vi "CAPFM-Acquire.vi"(0 "Runtime":T2, 11 "error in (no error)":errorcluster, 13 "Refs":T1) -> (6 "Control":dbl[](array[numeric]), 8 "Masked":dbl[](array[numeric]), 15 "error out":errorcluster)   [LabVIEW 2020]
uses:
  Typedefs/CAPFM-Runtime Data.ctl
  Typedefs/CAPFM-Control References.ctl
  <vilib>/Analysis/baseanly.llb/Mean (DBL).vi
  epl-vi-lib/Utility VIs/Conversion VIs/Create Waveform Cluster (2D).vi
  <vilib>/Analysis/NI_AALBase.lvlib
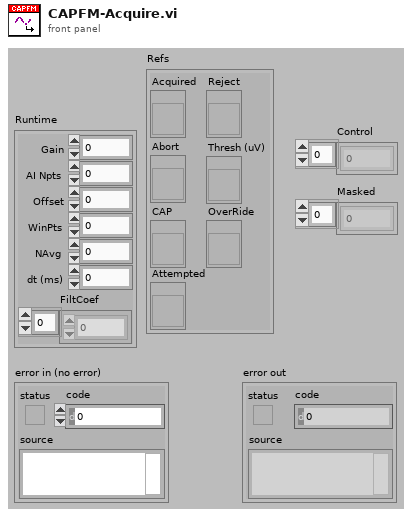
[diagram p1: front panel]
types:
  T1 = typedef "CAPFM-Control References.ctl" = cluster{"Acquired":refnum<vi>, "Abort":refnum<vi>, "CAP":refnum<vi>, "Reject":refnum<vi>, "Thresh (uV)":refnum<vi>, "OverRide":refnum<vi>, "Attempted":refnum<vi>}
  T2 = typedef "CAPFM-Runtime Data.ctl" = cluster{"Offset":i32, "AI Npts":i32, "Gain":dbl, "WinPts":i32, "NAvg":i32, "dt (ms)":dbl, "FiltCoef":dbl[]}
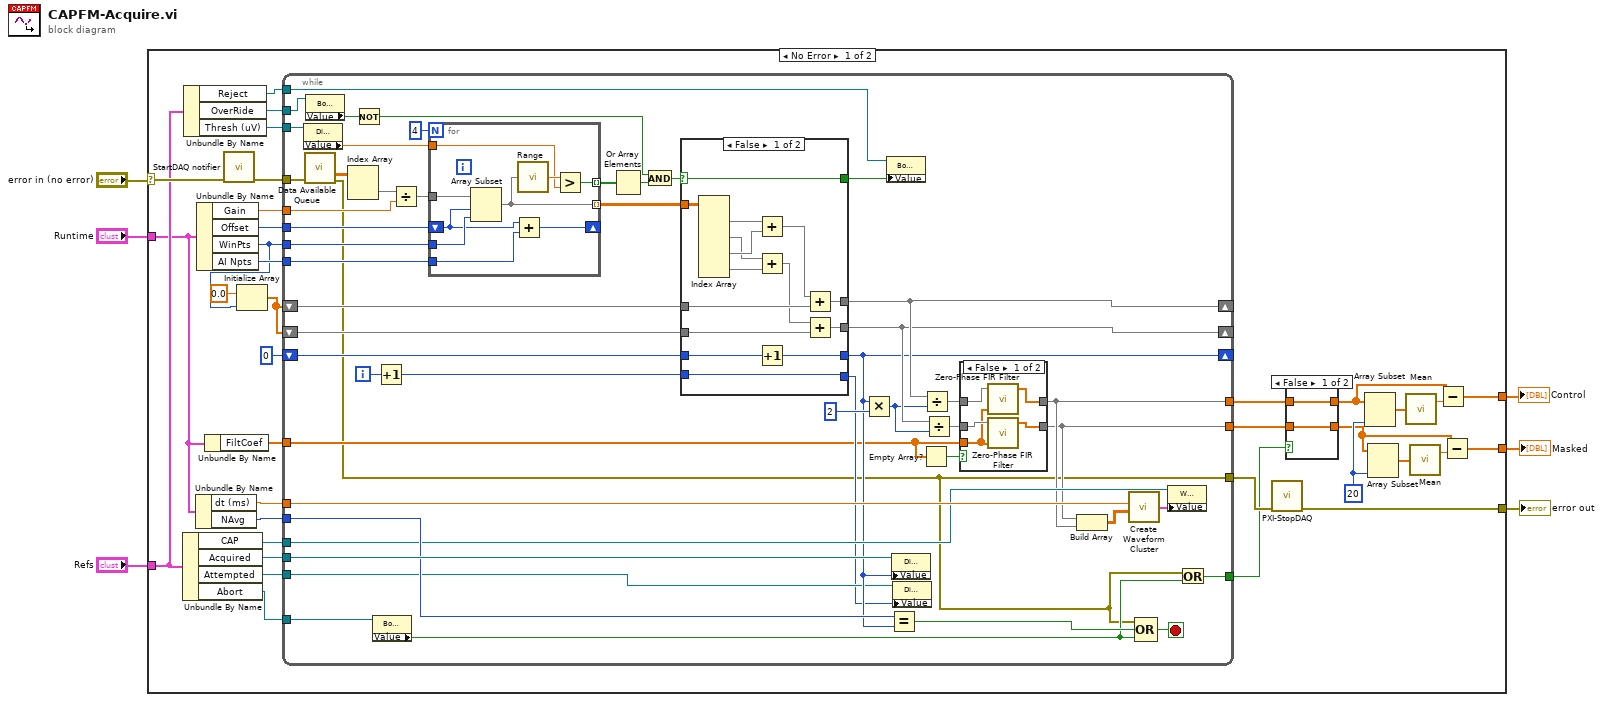
[diagram p0: block diagram]
diagram:
  n1 = case shown="No Error" "error in (no error)" {
    selector: "error in (no error)" -> [w41 w130]
    tunnel: [w29 w130] -> w5
    tunnel: "Runtime" -> [w8 _]
    tunnel: "Refs" -> [w22 _]
    tunnel: [w10 _] -> w2
    tunnel: [w9 _] -> w1
    frame No Error {
      w17 = 20
      n2 = Unbundle By Name(w22) -> ("CAP"=w31:refnum<vi>, "Acquired"=w35:refnum<vi>, "Attempted"=w19:refnum<vi>, "Abort"=w33:refnum<vi>)
      n3 = Unbundle By Name(w22) -> ("Reject"=w18:refnum<vi>, "OverRide"=w20:refnum<vi>, "Thresh (uV)"=w21:refnum<vi>)
      n4 = Unbundle By Name(w8) -> ("dt (ms)"=w32:dbl, "NAvg"=w34:i32)
      n5 = Unbundle By Name(w8) -> ("Gain"=w39:dbl, "Offset"=w37:i32, "WinPts"=w26:i32, "AI Npts"=w38:i32)
      n6 = Unbundle By Name(w8) -> ("FiltCoef"=w7:dbl[])
      n7 = call "StartDAQ notifier.vi"("error in (no error)"=w41) -> ("error out"=w40:errorcluster)  [unwired: 6 in]
      n8 = Initialize Array(0.0 ("element"), w26) -> (w28:dbl[])
      n9 = while {
        tunnel: w40 -> [w93]
        tunnel: w39 -> [w90]
        tunnel: w26 -> [w87]
        tunnel: w38 -> [w86]
        tunnel: w37 -> [w85]
        shift-right: [w75] -> _
        shift-left: w28 -> [w83]
        shift-right: [w74] -> _
        shift-left: w28 -> [w82]
        shift-right: [w57] -> _
        shift-left: 0 -> [w58]
        tunnel: w35 -> [w80]
        tunnel: w34 -> [w79]
        tunnel: w33 -> [w76]
        tunnel: w32 -> [w72]
        tunnel: w31 -> [w71]
        tunnel: [w46] -> w23
        tunnel: [w45] -> w24
        tunnel: [w44] -> w30
        tunnel: [w67] -> w25
        tunnel: w21 -> [w66]
        tunnel: w20 -> [w61]
        tunnel: w19 -> [w56]
        tunnel: w18 -> [w53]
        tunnel: w7 -> [w49]
        i -> [w55]
        stop <- w78 stop-if-true
        n10 = property class="DigNum (strict)"(reference=w66) -> ("Value"=w65:dbl)  [unwired: 1 in, 2 out]
        n11 = call "Data Available Queue.vi"("error in (no error)"=w93) -> ("AI Waveforms"=w92:dbl[][], "error out"=w44:errorcluster)  [unwired: 10 in, 3 out]
        n12 = property class="Bool (strict)"(reference=w61) -> ("Value"=w60:bool)  [unwired: 1 in, 2 out]
        n13 = Index Array(array=w92) -> (element=w91:dbl[])  [unwired: 2 in]
        n14 = Not(x=w60) -> (.not. x?=w59:bool)
        n15 = property class="Bool (strict)"(reference=w76) -> ("Value"=w68:bool)  [unwired: 1 in, 2 out]
        n16 = Increment(x=w55) -> (x+1=w52:i32)
        n17 = Divide(x=w91, y=w90) -> (x/y=w88:dbl[])
        n18 = for {
          N: 4 -> [_]
          tunnel: w88 -> [w129]
          shift-right: [w127] -> _
          shift-left: w85 -> [w126]
          tunnel: w87 -> [w128]
          tunnel: w86 -> [w125]
          tunnel: [w124] -> w84 mode=indexing
          tunnel: w65 -> [w122]
          tunnel: [w121] -> w64 mode=indexing
          n19 = Array Subset(array=w129, index=w126, length=w128) -> (w124:dbl[])
          n20 = Add(x=w126, y=w125) -> (x+y=w127:i32)
          n21 = call "Range.vi"("Array"=w124) -> ("Range"=w123:dbl)
          n22 = Greater?(x=w123, y=w122) -> (0:w121:bool)
        }
        n23 = Or Array Elements(Boolean array=w64) -> (logical OR=w63:bool)
        n24 = And(x=w59, y=w63) -> (x .and. y?=w62:bool)
        n25 = case shown="False" w62 {
          selector: w62 -> [w102 w117]
          tunnel: w84 -> [w115 _]
          tunnel: w83 -> [w109 w120]
          tunnel: w82 -> [w107 w119]
          tunnel: [w106 w120] -> w75
          tunnel: [w105 w119] -> w74
          tunnel: w58 -> [w104 w118]
          tunnel: [w103 w118] -> w57
          tunnel: [w102 w117] -> w54
          tunnel: [w101 w116] -> w51
          tunnel: w52 -> [w101 w116]
          frame False {
            n26 = Index Array(array=w115) -> (element #1=w114:dbl[], element #2=w111:dbl[], element #3=w113:dbl[], element #4=w112:dbl[])  [unwired: 8 in]
            n27 = Add(x=w114, y=w113) -> (x+y=w110:dbl[])
            n28 = Add(x=w111, y=w112) -> (x+y=w108:dbl[])
            n29 = Increment(x=w104) -> (x+1=w103:i32)
            n30 = Add(x=w110, y=w109) -> (x+y=w106:dbl[])
            n31 = Add(x=w108, y=w107) -> (x+y=w105:dbl[])
          }
          frame True {
          }
        }
        n32 = Multiply(x=w57, y=2) -> (x*y=w73:i32)
        n33 = property class="Bool (strict)"(reference=w53, "Value"=w54) -> ()  [unwired: 1 in, 2 out]
        n34 = Equal?(x=w79, y=w57) -> (x = y?=w77:bool)
        n35 = property class="DigNum (strict)"(reference=w80, "Value"=w57) -> ()  [unwired: 1 in, 2 out]
        n36 = property class="DigNum (strict)"(reference=w56, "Value"=w51) -> ()  [unwired: 1 in, 2 out]
        n37 = Empty Array?(array=w49) -> (empty?=w50:bool)
        n38 = Divide(x=w75, y=w73) -> (x/y=w48:dbl[])
        n39 = Divide(x=w74, y=w73) -> (x/y=w47:dbl[])
        n40 = case shown="False" w50 {
          tunnel: w49 -> [w94 _]
          tunnel: w48 -> [w98 w100]
          tunnel: w47 -> [w96 w99]
          tunnel: [w97 w100] -> w46
          tunnel: [w95 w99] -> w45
          frame False {
            n41 = call "Zero-Phase FIR Filter.vi"("FIR Windowed Coefficients"=w94, "Array"=w98) -> ("Filtered Array"=w97:dbl[])  [unwired: 3 in]
            n42 = call "Zero-Phase FIR Filter.vi"("FIR Windowed Coefficients"=w94, "Array"=w96) -> ("Filtered Array"=w95:dbl[])  [unwired: 3 in]
          }
          frame True {
          }
        }
        n43 = Build Array(w45, w46) -> (w70:dbl[][])
        n44 = call-poly "Create Waveform Cluster.vi"("dx"=w72, "Array"=w70) -> ("waveform cluster"=w69:cluster{"offset":dbl, "dx":dbl, "Y":dbl[][]})  [unwired: 3 in]
        n45 = Compound Arithmetic op=OR(w44, w77, w68) -> (w78:bool)
        n46 = property class="WFGraph (strict)"(reference=w71, "Value"=w69) -> ()  [unwired: 1 in, 2 out]
        n47 = Or(x=w44, y=w68) -> (x .or. y?=w67:bool)
      }
      n48 = call "PXI-StopDAQ.vi"("error in (no error)"=w30) -> ("error out"=w29:errorcluster)  [unwired: 6 in]
      n49 = case shown="False" w25 {
        tunnel: [w43 _] -> w11
        tunnel: w24 -> [w43 _]
        tunnel: w23 -> [w42 _]
        tunnel: [w42 _] -> w12
        frame False {
        }
        frame True {
        }
      }
      n50 = Array Subset(array=w12, length=w17) -> (w15:dbl[])  [unwired: 1 in]
      n51 = Array Subset(array=w11, length=w17) -> (w16:dbl[])  [unwired: 1 in]
      n52 = call-poly <vilib>:"Mean.vi"("X"=w15) -> ("mean"=w14:dbl)  [unwired: 1 out]
      n53 = call-poly <vilib>:"Mean.vi"("X"=w16) -> ("mean"=w13:dbl)  [unwired: 1 out]
      n54 = Subtract(x=w12, y=w14) -> (x-y=w10:dbl[])
      n55 = Subtract(x=w11, y=w13) -> (x-y=w9:dbl[])
    }
    frame Error {
    }
  }
  "error out" <- w5
  "Control" <- w2
  "Masked" <- w1
